vi "Test WebService.vi"() -> ()   [LabVIEW 2020]
uses:
  <vilib>/httpClient/POSTBuffer.vi
  <vilib>/httpClient/LabVIEWHTTPClient.lvlib
panel:
  out "body 2":string
  out "error out 2":errorcluster
  out "error out":errorcluster
  out "body":string
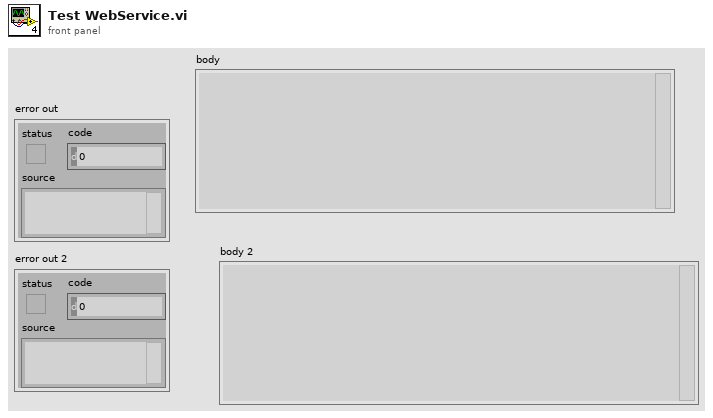
[diagram p1: front panel]
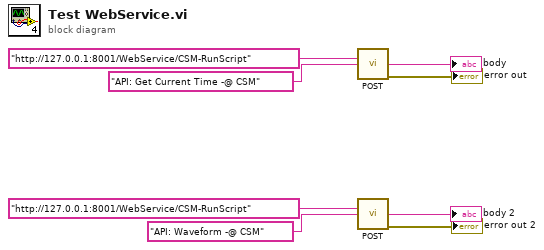
[diagram p0: block diagram]
diagram:
  n1 = call-poly <vilib>:"POST.vi"("url"="http://127.0.0.1:8001/WebService/CSM-RunScript" ("buffer"), "buffer"="API: Get Current Time -@ CSM") -> ("body"=→"body":string, "error out"=→"error out":errorcluster)  [unwired: 10 in, 2 out]
  n2 = call-poly <vilib>:"POST.vi"("url"="http://127.0.0.1:8001/WebService/CSM-RunScript" ("buffer"), "buffer"="API: Waveform -@ CSM") -> ("body"=→"body 2":string, "error out"=→"error out 2":errorcluster)  [unwired: 10 in, 2 out]
